vi "imageTobase64.vi"(8 "error in (no error)":errorcluster, 11 "path to PNG file":path) -> (0 "error out":errorcluster, 3 "string out (base64-encoded)":string)   [LabVIEW 2011]
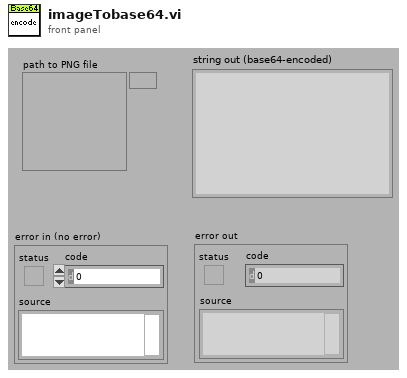
[diagram p1: front panel]
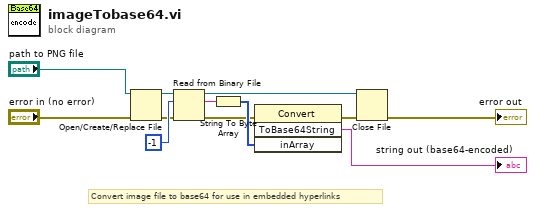
[diagram p0: block diagram]
diagram:
  # "Convert image file to base64 for use in embedded hyperlinks"
  n1 = Open/Create/Replace File(file path (use dialog)="path to PNG file", error in="error in (no error)") -> (refnum out=w9:refnum<file>, error out=w1:errorcluster)  [unwired: 4 in, 1 out]
  n2 = Read from Binary File(8:w1, 10:-1 ("count (1)"), 11:w9) -> (0:w3:errorcluster, 2:w7:string, 3:w4:refnum<file>)  [unwired: 3 in, 1 out]
  n3 = String To Byte Array(string=w7) -> (unsigned byte array=w10:u8[])
  n4 = invoke class="Convert" method="ToBase64String"(error in=w3, "inArray"=w10) -> (error out=w6:errorcluster, "ToBase64String"=→"string out (base64-encoded)":string)  [unwired: 2 in, 2 out]
  n5 = Close File(refnum=w4, error in=w6) -> (error out=→"error out":errorcluster)  [unwired: 1 out]
